vi "Savitsky Golay Filter (multiple).vi"(8 "error in (no error)":errorcluster, 10 "side points":i32, 11 "XY-data":cluster{"X-array":dbl[], "Y-array":dbl[]}[](array[cluster])) -> (0 "error out":errorcluster, 3 "XY-data out":cluster{"X-array":dbl[], "Y-array":dbl[]}[](array[cluster]) {"Y-array" format="%.2p"; "X-array" format="%.2p"})   [LabVIEW 2019, in "xy_utilities.lvlib"]
doc: "Filter <b>XY-data</b>'s Y-Array with a Savitsky-Golay FIR smoothing filter.\n\n<b>side points</b> specifies the number of data points to each side of the current data point to use for the least squares minimization. side points*2 + 1 is the length of the moving window, which must be greater than the polynomial order.\n\nWire data to the data input to determine the polymorphic instance to use or manually select the instance."
uses:
  xy_utilities.lvlib
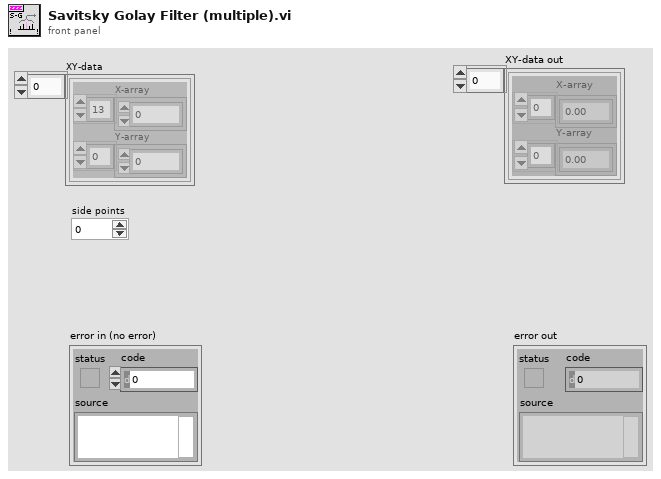
[diagram p1: front panel]
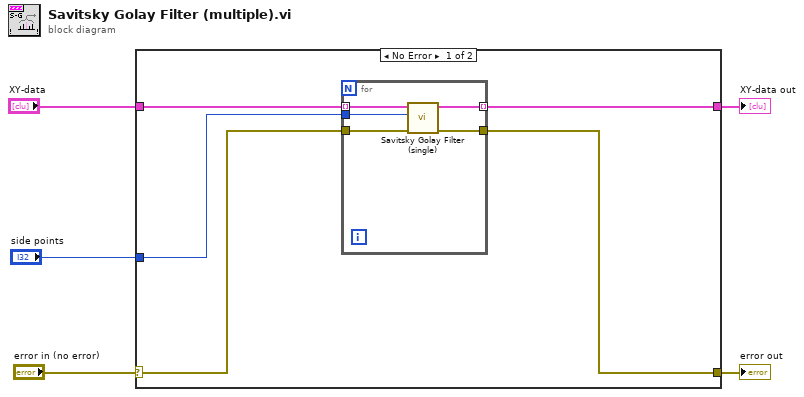
[diagram p0: block diagram]
diagram:
  n1 = case shown="No Error" "error in (no error)" {
    selector: "error in (no error)" -> [w7 w17]
    tunnel: [w6 w17] -> w4
    tunnel: "XY-data" -> [w10 w16]
    tunnel: [w9 w16] -> w2
    tunnel: "side points" -> [w8 _]
    frame No Error {
      n2 = for {
        tunnel: w10 -> [w15] mode=indexing
        tunnel: [w14] -> w9 mode=indexing
        tunnel: w8 -> [w13]
        tunnel: w7 -> [w12]
        tunnel: [w11] -> w6
        n3 = call "Savitsky Golay Filter (single).vi"("error in (no error)"=w12, "side points"=w13, "XY-data"=w15) -> ("error out"=w11:errorcluster, "XY-data out"=w14:cluster{"X-array":dbl[], "Y-array":dbl[]})  [unwired: 7 in]
      }
    }
    frame Error {
    }
  }
  "error out" <- w4
  "XY-data out" <- w2
